vi "ClearLastError.vi"(7 "DLL path":path, 8 "error in (no error)":errorcluster, 11 "session id in":i32) -> (0 "error out":errorcluster, 3 "session id out":i32)   [LabVIEW 2017, in "ONNX Class Library.lvlib"]
doc: "/**\n * @brief Очистить сообщение об ошибке для сессии\n * \n * Сбрасывает сохраненное сообщение об ошибке. Полезно после обработки ошибки,\n * чтобы не получить старое сообщение при следующей проверке.\n * \n * @param sessionId [IN] ID сессии\n * \n * @return void\n */\nvoid ClearLastError(int sessionId);"
uses:
  ONNX Class Library.lvlib
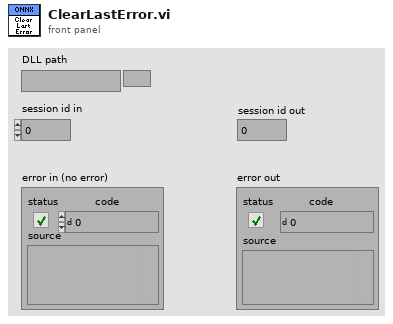
[diagram p1: front panel]
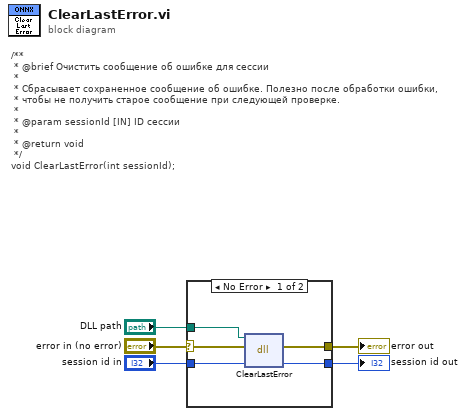
[diagram p0: block diagram]
diagram:
  # "/**\n * @brief Очистить сообщение об ошибке для сессии\n * \n * Сбрасывает сохраненное сообщение об ошибке. Полезно после обработки ошибки,\n * чтобы не получить старое сообщение при следующей проверке.\n * \n * @param sessionId [IN] ID сессии\n * \n * @return void\n */\nvoid ClearLastError(int sessionId);"
  n1 = case shown="No Error" "error in (no error)" {
    selector: "error in (no error)" -> [w6 w12]
    tunnel: [w10 w12] -> w5
    tunnel: "session id in" -> [w9 w11]
    tunnel: [w8 w11] -> w3
    tunnel: "DLL path" -> [w7 _]
    frame No Error {
      n2 = dll-call lib="home/ivan/LabVIEWData/ONNX/Test/libonnx_wrapper/unix64/libonnx_wrapper.so" fn="ClearLastError"(path in=w7, error in=w6, "sessionId"=w9) -> (error out=w10:errorcluster, "sessionId"=w8:i32)  [unwired: 2 in, 1 out]
    }
    frame Error {
    }
  }
  "error out" <- w5
  "session id out" <- w3
